vi "Create Default Values 90.vi"() -> ()   [LabVIEW 2014]
panel:
  in  "LabVIEW._Application":refnum<k7>
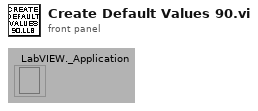
[diagram p1: front panel]
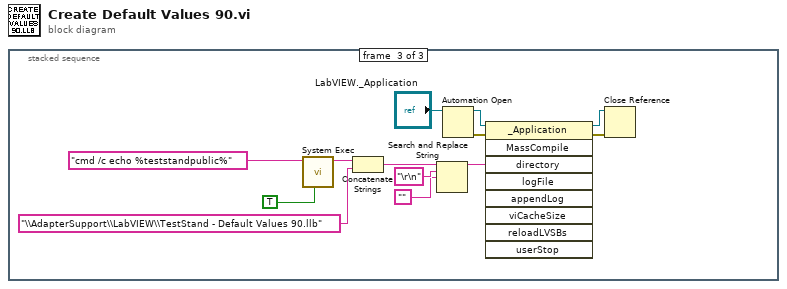
[diagram p0: block diagram]
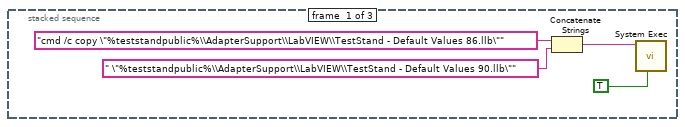
[diagram p2: hidden frame]
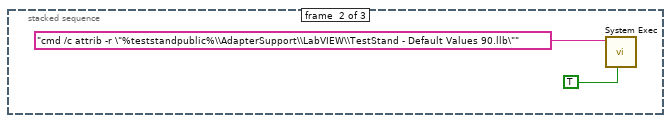
[diagram p3: hidden frame]
diagram:
  n1 = stacked-sequence {
    frame #0 {
      n2 = Concatenate Strings("cmd /c copy \"%teststandpublic%\\AdapterSupport\\LabVIEW\\TestStand - Default Values 86.llb\"" ("command line"), " \"%teststandpublic%\\AdapterSupport\\LabVIEW\\TestStand - Default Values 90.llb\"" ("command line")) -> (w2:string)
      n3 = call <vilib>:"System Exec.vi"("run minimized? (F)"=TRUE, "command line"=w2) -> ()  [unwired: 6 in, 4 out]
    }
    frame #1 {
      n4 = call <vilib>:"System Exec.vi"("run minimized? (F)"=TRUE, "command line"="cmd /c attrib -r \"%teststandpublic%\\AdapterSupport\\LabVIEW\\TestStand - Default Values 90.llb\"") -> ()  [unwired: 6 in, 4 out]
    }
    frame #2 {
      n5 = call <vilib>:"System Exec.vi"("run minimized? (F)"=TRUE, "command line"="cmd /c echo %teststandpublic%") -> ("standard output"=w7:string)  [unwired: 6 in, 3 out]
      n6 = Concatenate Strings(w7, "\\AdapterSupport\\LabVIEW\\TestStand - Default Values 90.llb" ("string")) -> (w13:string)
      n7 = Search and Replace String(input string=w13, search string="\r\n", replace string="") -> (result string=w10:string)  [unwired: 5 in, 3 out]
      n8 = Automation Open(Automation Refnum="LabVIEW._Application") -> (Automation Refnum=w18:refnum<k7>, error out=w17:errorcluster)  [unwired: 3 in]
      n9 = invoke class="_Application" method="MassCompile"(reference=w18, error in=w17, "directory"=w10) -> (reference out=w15:refnum<k7>, error out=w14:errorcluster)  [unwired: 6 in, 7 out]
      n10 = Close Reference(reference=w15, error in (no error)=w14) -> ()  [unwired: 1 out]
    }
  }
